vi "checkBeginBallPlacementAllyPlay.vi"(8 "error in (no error)":errorcluster, 10 "Referee":refnum<class "Referee.lvclass">, 11 "BallPlacementAllyPlay in":refnum<class "BallPlacementAllyPlay.lvclass">) -> (0 "error out":errorcluster, 2 "BeginBallPlacementAlly":bool, 3 "BallPlacementAllyPlay out":refnum<class "BallPlacementAllyPlay.lvclass">)   [LabVIEW 2020, in "BallPlacementAllyPlay.lvclass"]
uses:
  BallPlacementAllyPlay.lvclass
  Referee_class/Referee.lvclass
  Referee_class/command_interpreted.ctl
  Referee_class/Referee.lvclass/Referee.ctl
  Referee_class/Read command_interpreted.vi
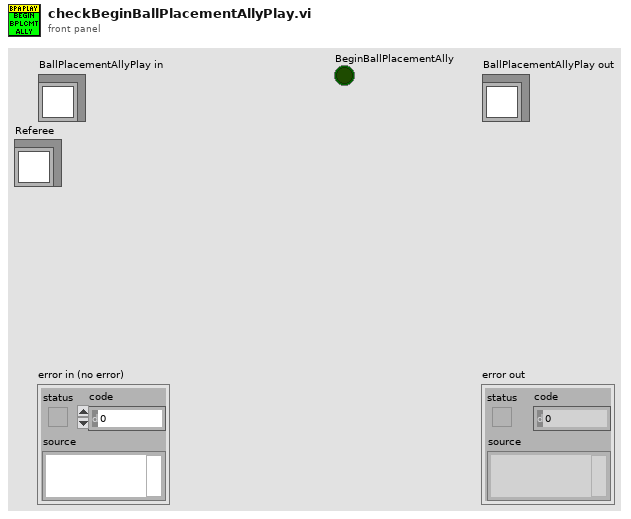
[diagram p1: front panel]
types:
  T1 = typedef "command_interpreted.ctl" = enum16{"Goal Ally", "Goal Enemy", "Ball Placement Enemy", "Ball Placement Ally", "Normal Half Time", "Extra Time  Break", "Extra Half Time", "None", "Post Game", "PKA Normal Start", "Prepare Kickoff Ally", "PKE Normal Start", "Prepare Kickoff Enemy", "Force Start", "Halt", "Timeout", "Prepare Penalty Ally", "Prepare Penalty Enemy", "PPA NormalStart", "PPE Normal Start", "Indirect Free Ally", "Direct Free Enemy", "Direct Free Ally", "Indirect Free Enemy", "Stop"}
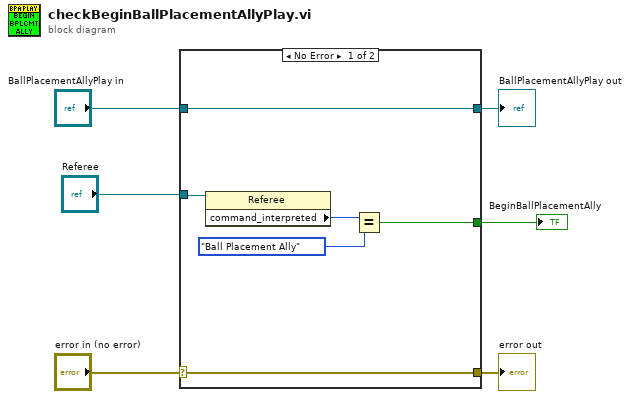
[diagram p0: block diagram]
diagram:
  n1 = case shown="No Error" "error in (no error)" {
    selector: "error in (no error)" -> [w11 w14]
    tunnel: [w11 w14] -> w5
    tunnel: [w12 w13] -> w3
    tunnel: "BallPlacementAllyPlay in" -> [w12 w13]
    tunnel: "Referee" -> [w10 _]
    tunnel: [w7 _] -> w1
    frame No Error {
      n2 = property class="Referee"(reference=w10) -> ("command_interpreted"=w9:T1)  [unwired: 1 in, 2 out]
      n3 = Equal?(x=w9, y=command_interpreted."Ball Placement Ally") -> (x = y?=w7:bool)
    }
    frame Error {
    }
  }
  "error out" <- w5
  "BallPlacementAllyPlay out" <- w3
  "BeginBallPlacementAlly" <- w1
